vi "0_5V_converter.vi"(1 "Target Low":dbl format="%#_13g", 2 "Source":dbl[](array[numeric]) format="%#_13g", 3 "Target High":dbl format="%#_13g") -> (0 "Target":dbl[](array[numeric]) format="%#_13g")   [LabVIEW 2017, in "sensor_translation.lvlib"]
uses:
  sensor_translation.lvlib
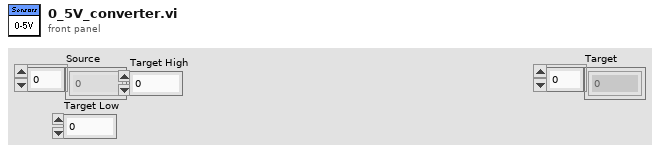
[diagram p1: front panel]
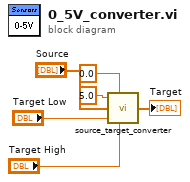
[diagram p0: block diagram]
diagram:
  n1 = call "source_target_converter.vi"("Source High"=5.0, "Source Low"=0.0, "Source"="Source", "Target Low"="Target Low", "Target High"="Target High") -> ("Target"=→"Target":dbl[])
